vi "Measurement Template(Stream).vi"(8 "error in (no error)":errorcluster, 10 "stop":bool, 11 "measurement configuration":cluster{"Boolean":bool}) -> (0 "error out":errorcluster, 3 "measurement results":cluster{"Boolean":bool})   [LabVIEW 2021]
uses:
  Runtime/Clients/Measurement Service Client V2/RPC Messages/ni_measurementlink_measurement_v2_MeasureRequest.ctl
  Runtime/Clients/Measurement Service Client V2/RPC Messages/google_protobuf_Any.ctl
  Runtime/Clients/Measurement Service Client V2/RPC Messages/ni_measurementlink_PinMapContext.ctl
  35f71eb9-7158-4110-bfb1-6d749e6fa8f4.vi
  ef0035e8-05ef-469b-9be2-5e457b1f40d8.vi
  <vilib>/gRPC/LabVIEW gRPC Library/Server API/Translate Protobuf Error.vi
  <vilib>/AdvancedString/1D String Array to Delimited String.vi
  <vilib>/gRPC/LabVIEW gRPC Library/Server API/Server/Get Server DLL Path.vi
  <vilib>/gRPC/LabVIEW gRPC Library/grpc-lvsupport-release.lvlib
  Runtime/Clients/Measurement Service Client V2/Measurement Service Client V2.lvlib
  Runtime/Clients/Measurement Client V2/Client.lvlib
panel:
  in  "service class":string="Voltage Measurement_LabVIEW"
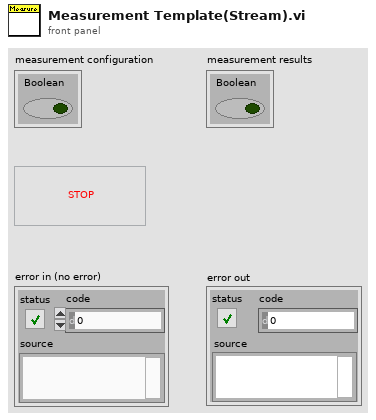
[diagram p1: front panel]
types:
  T1 = typedef "Measurement Service Client V2.lvlib/ni_measurementlink_measurement_v2_MeasureRequest.ctl" = cluster{"configuration_parameters":T2, "pin_map_context":T3}
  T2 = typedef "Measurement Service Client V2.lvlib/google_protobuf_Any.ctl" = cluster{"type_url":string, "value":u8[]}
  T3 = typedef "Measurement Service Client V2.lvlib/ni_measurementlink_PinMapContext.ctl" = cluster{"pin_map_id":string, "sites":i32[]}
  T4 = typedef "grpc-lvsupport-release.lvlib/grpcId.ctl" = u64
  T5 = typedef "grpc-lvsupport-release.lvlib/Message Metadata.ctl" = cluster{"Version":i32, "Name":string, "Type Url":string, "Elements":T6[], "Has Oneof":bool}
  T6 = typedef "grpc-lvsupport-release.lvlib/Message Element Metadata.ctl" = cluster{"Field Name":string, "Embedded Message Name":string, "Protobuf Index":i32, "MessageElementType":T7, "Repeated":bool, "Is in Oneof":bool, "Oneof Container Name":string}
  T7 = typedef "grpc-lvsupport-release.lvlib/Message Element Type.ctl" = enum32{"Int32Value", "FloatValue", "DoubleValue", "BoolValue", "StringValue", "MessageValue", "Int64Value", "UInt32Value", "UInt64Value", "EnumValue", "Bytes", "Fixed64", "Fixed32", "SFixed64", "SFixed32", "SInt64", "SInt32"}
  T8 = typedef "grpc-lvsupport-release.lvlib/Any.ctl" = cluster{"Type Url":string, "Bytes":u8[]}
  T9 = typedef "Measurement Service Client V2.lvlib/ni_measurementlink_measurement_v2_MeasureResponse.ctl" = cluster{"outputs":T2}
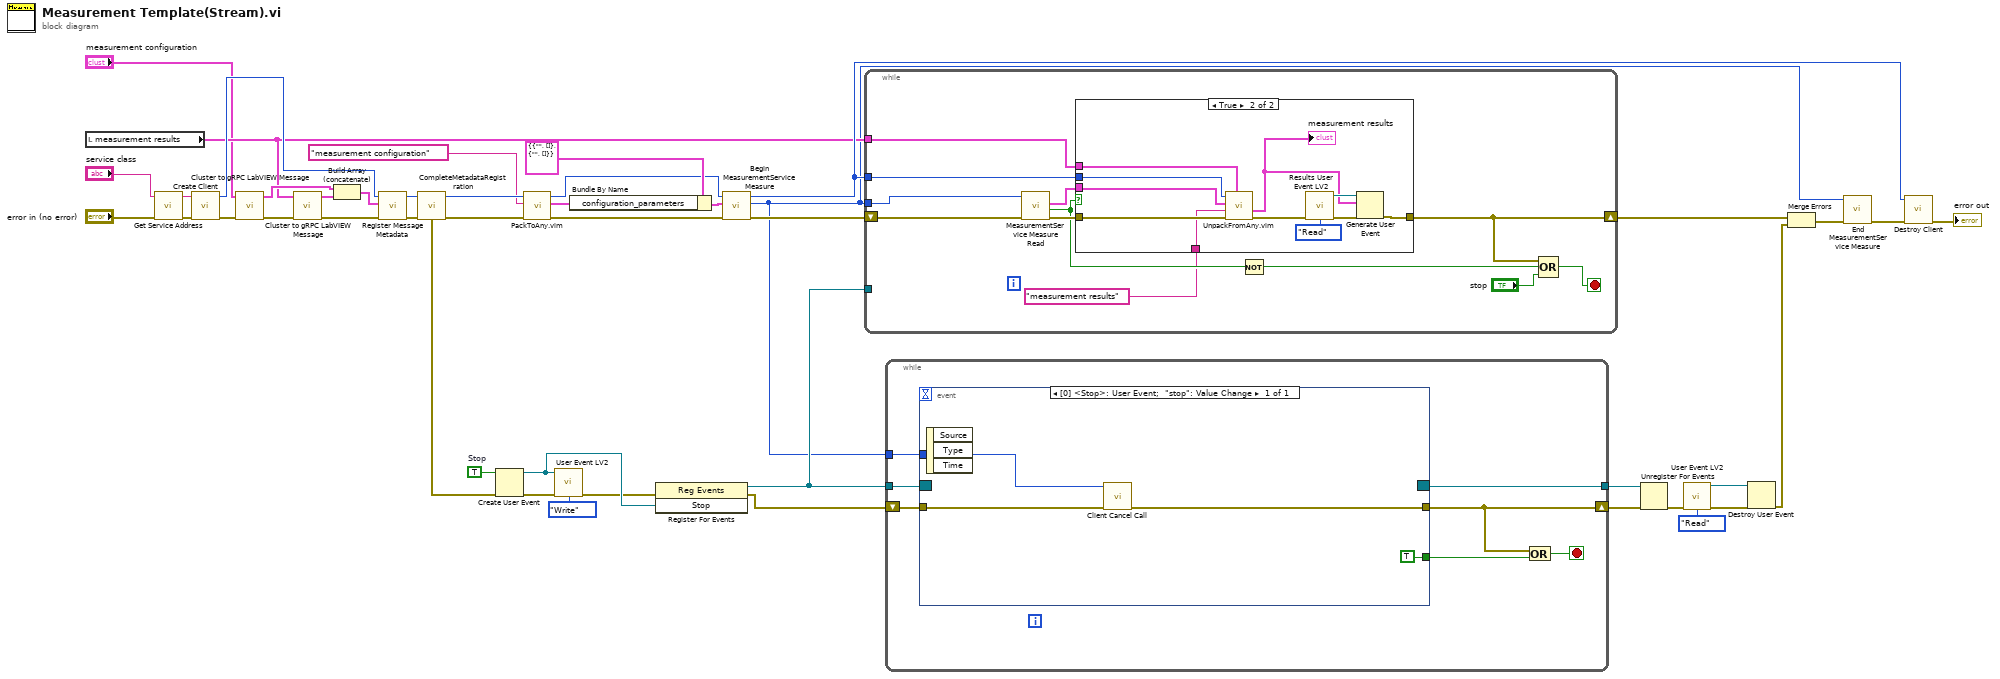
[diagram p0: block diagram]
diagram:
  w19 = TRUE  # Stop
  n1 = local read "measurement results"() -> (w22:cluster{"Boolean":bool})
  n2 = call "Get Service Address.vi"("error in"="error in (no error)", "service to run"="service class") -> ("error out"=w34:errorcluster, "service address"=w32:string)  [unwired: 8 in]
  n3 = call "Create Client.vi"("error in"=w34, "address"=w32) -> ("error out"=w31:errorcluster, "gRPC ID Out"=w30:T4)  [unwired: 8 in]
  n4 = call <vilib>:"Cluster to gRPC LabVIEW Message.vi"("error in"=w31, "Cluster"="measurement configuration") -> ("error out"=w36:errorcluster, "gRPC Message Metadata []"=w44:T5[])  [unwired: 7 in, 1 out]
  n5 = call <vilib>:"Cluster to gRPC LabVIEW Message.vi"("error in"=w36, "Cluster"=w22) -> ("error out"=w35:errorcluster, "gRPC Message Metadata []"=w43:T5[])  [unwired: 7 in, 1 out]
  n6 = Build Array (concatenate)(w44, w43) -> (w42:T5[])
  n7 = call <vilib>:"Register Message Metadata.vi"("error in"=w35, "Messages"=w42, "gRPCid in"=w30) -> ("error out"=w41:errorcluster, "gRPCid out"=w29:T4)  [unwired: 7 in]
  n8 = call <vilib>:"CompleteMetadataRegistration.vi"("error in"=w41, "gRPC ID in"=w29) -> ("error out"=w18:errorcluster, "gRPC ID Out"=w28:T4)  [unwired: 8 in]
  n9 = Create User Event(user event datatype=w19, error in=w18) -> (user event=w15:refnum<user-event>, error out=w13:errorcluster)
  n10 = call "PackToAny.vim"("error in"=w18, "Message Type"="measurement configuration", "gRPCid in"=w28) -> ("error out"=w40:errorcluster, "Any"=w38:T8, "gRPCid out"=w24:u64)  [unwired: 6 in]
  n11 = call "User Event LV2.vi"("Stop event"=w15, "error in (no error)"=w13, "LV2 operations"=enum16{"Read", "Write"}."Write") -> ("error out"=w14:errorcluster)  [unwired: 11 in, 1 out]
  n12 = Bundle By Name(cluster=T1 {"configuration_parameters"={"type_url"="", "value"=[]}, "pin_map_context"={"pin_map_id"="", "sites"=[]}} ("Request Data"), "configuration_parameters"=w38) -> (w37:T1)
  n13 = register-events(error in=w14, w15) -> (reference out=w8:refnum<event-registration>, error out=w7:errorcluster)  [unwired: 1 in]
  n14 = call "Begin MeasurementService Measure.vi"("error in"=w40, "Request Data"=w37, "gRPC ID"=w24) -> ("error out"=w17:errorcluster, "Call Id Out"=w1:T4, "gRPC ID out"=w25:T4)  [unwired: 6 in]
  n15 = while {
    tunnel: w1 -> [w55]
    tunnel: w25 -> [w54]
    shift-right: [w52] -> w4
    shift-left: w17 -> [w56]
    tunnel: w22 -> [w53]
    tunnel: w8 -> [_]
    stop <- w49 stop-if-true
    n16 = call "MeasurementService Measure Read.vi"("error in"=w56, "Call ID in"=w55) -> ("error out"=w47:errorcluster, "Success"=w46:bool, "Response Data"=w48:T9)  [unwired: 6 in, 1 out]
    n17 = case shown="True" w46 {
      tunnel: w48 -> [_ w68]
      tunnel: w54 -> [_ w67]
      tunnel: w47 -> [w57 w66]
      tunnel: [w57 w62] -> w52
      tunnel: w53 -> [_ w65]
      tunnel: "measurement results" ("Message Type") -> [_ w64]
      frame False {
      }
      frame True {
        n18 = call "UnpackFromAny.vim"("Data Type"=w65, "error in"=w66, "Message Type"=w64, "Any"=w68, "gRPCid in"=w67) -> ("error out"=w63:errorcluster, "Unpacked Value"=w59:cluster{"Boolean":bool})  [unwired: 4 in, 1 out]
        "measurement results" <- w59
        n19 = call "Results User Event LV2.vi"("error in (no error)"=w63, "LV2 operations"=enum16{"Read", "Write"}."Read") -> ("user event out"=w60:refnum<user-event>, "error out"=w61:errorcluster)  [unwired: 12 in]
        n20 = Generate User Event(user event=w60, event data cluster=w59, error in=w61) -> (error out=w62:errorcluster)  [unwired: 1 in, 1 out]
      }
    }
    n21 = Not(x=w46) -> (.not. x?=w50:bool)
    n22 = Compound Arithmetic op=OR(w52, w50, "stop") -> (w49:bool)
  }
  n23 = while {
    shift-right: [w74] -> w6
    shift-left: w7 -> [w75]
    tunnel: [w72] -> w5
    tunnel: w8 -> [w70]
    tunnel: w1 -> [w69]
    stop <- w71 stop-if-true
    n24 = event shown="[0] <Stop>: User Event;  \"stop\": Value Change" {
      selector: w70 -> [_]
      dyn-events: [_] -> w72
      timeout: _ -> [_]
      tunnel: w75 -> [w79]
      tunnel: [w78] -> w74
      tunnel: [TRUE] -> w73
      tunnel: w69 -> [w76]
      event User Event; "stop": Value Change {
        n25 = event-data() -> ()  [unwired: 1 in, 3 out]
        n26 = call <vilib>:"Client Cancel Call.vi"("error in"=w79, "Call ID in"=w76) -> ("error out"=w78:errorcluster)  [unwired: 7 in, 2 out]
      }
    }
    n27 = Compound Arithmetic op=OR(w74, w73) -> (w71:bool)
  }
  n28 = Unregister For Events(event registration refnum=w5, error in=w6) -> (error out=w9:errorcluster)
  n29 = call "User Event LV2.vi"("error in (no error)"=w9, "LV2 operations"=enum16{"Read", "Write"}."Read") -> ("Stop event out"=w11:refnum<user-event>, "error out"=w10:errorcluster)  [unwired: 12 in]
  n30 = Destroy User Event(user event=w11, error in=w10) -> (error out=w2:errorcluster)
  n31 = Merge Errors(w4, w2) -> (w3:errorcluster)
  n32 = call "End MeasurementService Measure.vi"("error in"=w3, "Call ID in"=w1) -> ("error out"=w26:errorcluster)  [unwired: 8 in, 1 out]
  n33 = call "Destroy Client.vi"("error in"=w26, "gRPC ID"=w25) -> ("error out"=→"error out":errorcluster)  [unwired: 9 in]
